vi "init_infoGet.vi"(5 "error in (no error)":errorcluster, 7 "spectrIdx":u16) -> (15 "serialNr":string, 17 "waveNrMin":sgl format="%.2f", 18 "waveNrMax":sgl format="%.2f", 19 "error out":errorcluster)   [LabVIEW 2010, in "OSA.lvclass"]
doc: "Lower level init routine."
uses:
  OSA.lvclass
  FTSLib.dll
panel:
  in  "serialNr dummy":string="1234567"
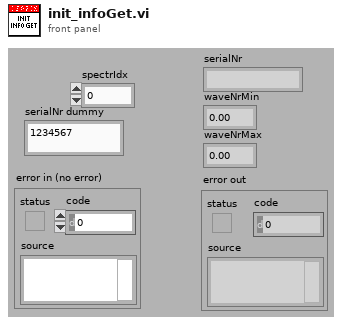
[diagram p1: front panel]
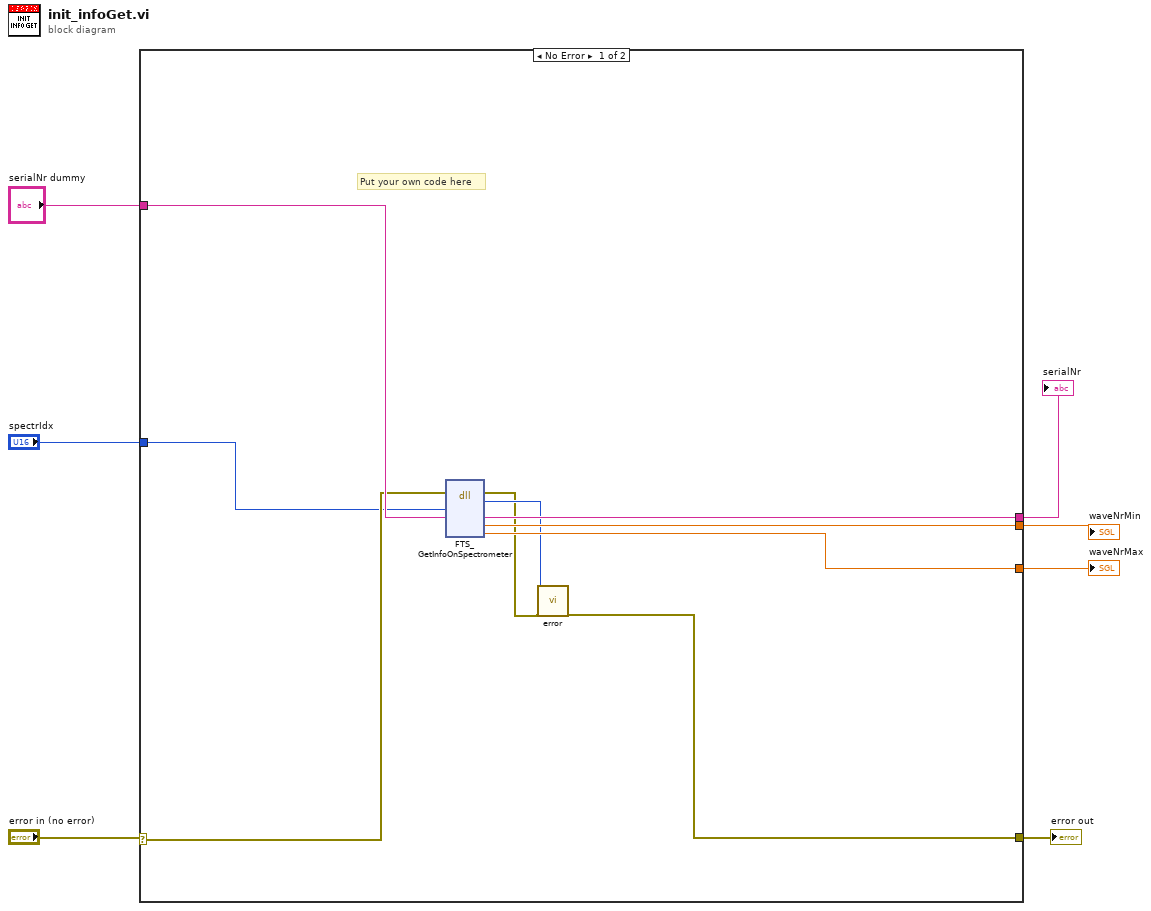
[diagram p0: block diagram]
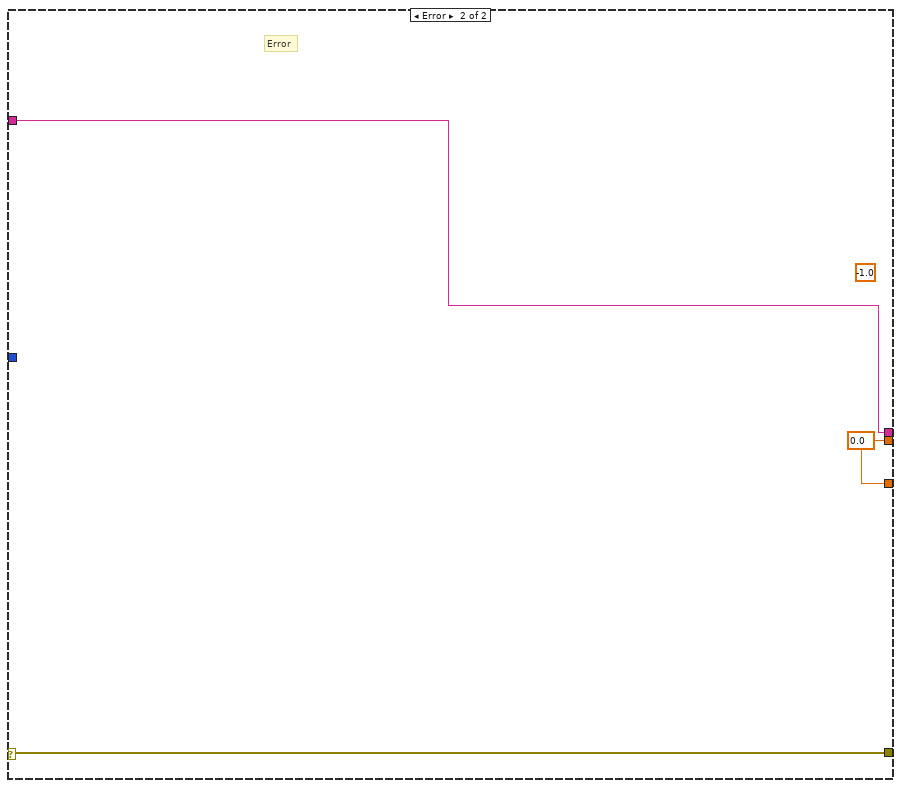
[diagram p2: hidden frame]
diagram:
  n1 = case shown="No Error" "error in (no error)" {
    selector: "error in (no error)" -> [w12 w19]
    tunnel: [w10 w19] -> w7
    tunnel: "spectrIdx" -> [w11 _]
    tunnel: [w16 w18] -> w4
    tunnel: [w15 w17] -> w3
    tunnel: [w14 w17] -> w2
    tunnel: "serialNr dummy" -> [w13 w18]
    frame No Error {
      # "Put your own code here"
      n2 = dll-call lib="FTSLib.dll" fn="FTS_GetInfoOnSpectrometer"(error in=w12, "spectrIdx"=w11, "serialNr"=w13) -> (error out=w8:errorcluster, "return type"=w9:i32, "serialNr"=w16:string, "waveNrMin"=w15:sgl, "waveNrMax"=w14:sgl)  [unwired: 5 in, 1 out]
      n3 = call "error.vi"("result code"=w9, "error in (no error)"=w8) -> ("error out"=w10:errorcluster)  [unwired: 15 in, 2 out]
    }
    frame Error {
      (unwired) -1.0 ("return type")
      w17 = sgl 0.0 ("waveNrMin")
      # "Error"
    }
  }
  "error out" <- w7
  "serialNr" <- w4
  "waveNrMin" <- w3
  "waveNrMax" <- w2
